vi "GlobalDataNum7.vi"(2 "Data  Numbers In":dbl[](array[numeric]), 3 "Data Number In":dbl, 4 "Element #":u16, 5 "Function select":string) -> (0 "Data Numbers Out":dbl[](array[numeric]), 1 "Data Number Out":dbl)   [LabVIEW 2013]
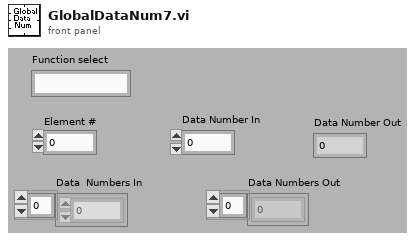
[diagram p1: front panel]
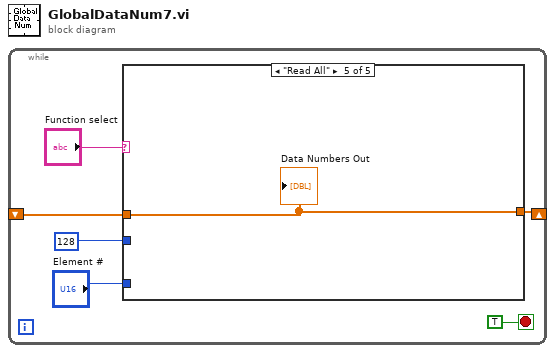
[diagram p0: block diagram]
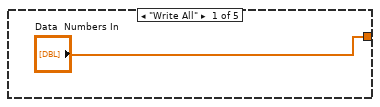
[diagram p2: hidden frame]
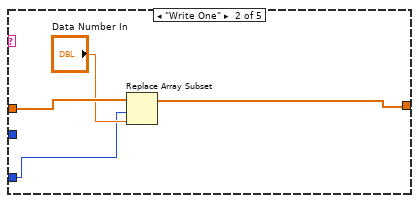
[diagram p3: hidden frame]
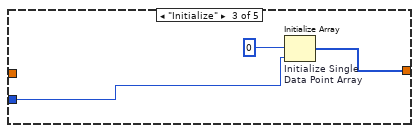
[diagram p4: hidden frame]
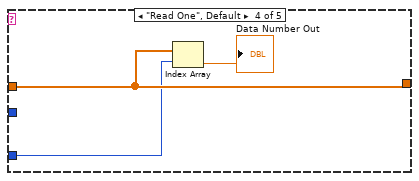
[diagram p5: hidden frame]
diagram:
  n1 = while {
    shift-right: [w4] -> _
    shift-left: _ -> [w3]
    stop <- TRUE stop-if-true
    n2 = case shown="\"Read All\"" "Function select" {
      tunnel: 128 -> [_ _ w14 _ _]
      tunnel: ["Data  Numbers In" w10 w13 w16 w18] -> w4
      tunnel: w3 -> [_ w11 _ w16 w18]
      tunnel: "Element #" -> [_ w8 _ w15 _]
      frame "Write All" {
      }
      frame "Write One" {
        n3 = Replace Array Subset(array=w11, new element="Data Number In", index=w8) -> (w10:dbl[])
      }
      frame "Initialize" {
        n4 = Initialize Array "Initialize Single\nData Point Array"(0, w14) -> (w13:i32[])
      }
      frame "Read One", Default {
        n5 = Index Array(array=w16, index=w15) -> (element=→"Data Number Out":dbl)
      }
      frame "Read All" {
        "Data Numbers Out" <- w18
      }
    }
  }
